vi "Initialize.vi"(8 "error in (no error)":errorcluster, 11 "FSR AI Channel":tag) -> (0 "error out":errorcluster, 3 "FSR":refnum<class "FSR.lvclass">)   [LabVIEW 2013, in "SGDV_Ctrl_v13_lib.lvlib" / "FSR.lvclass"]
uses:
  FSR.lvclass
  FSR.lvclass/FSR.ctl
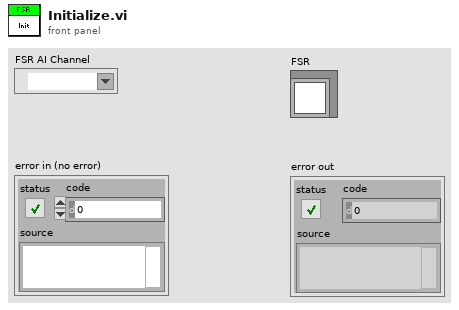
[diagram p1: front panel]
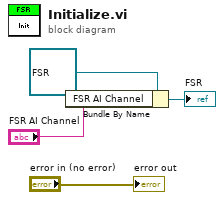
[diagram p0: block diagram]
diagram:
  n1 = Bundle By Name(cluster=refnum<class "FSR.lvclass"> refnum ("SGDV_Ctrl_v13_lib.lvlib:FSR.lvclass"), "FSR AI Channel"="FSR AI Channel") -> (→"FSR":refnum<class "FSR.lvclass">)
  "error out" <- "error in (no error)"
